vi "Increment Next Column.vi"(11 "SQL Statement in":refnum<class "SQL Statement.lvclass">) -> (3 "SQL Statement out":refnum<class "SQL Statement.lvclass">)   [LabVIEW 2013, in "SQLiteSupport.lvlib" / "SQL Statement.lvclass"]
uses:
  SQL Statement.lvclass
  SQL Statement.lvclass/SQL Statement.ctl
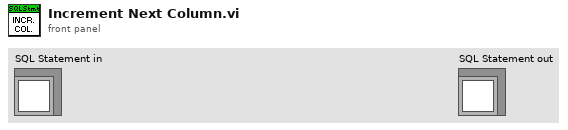
[diagram p1: front panel]
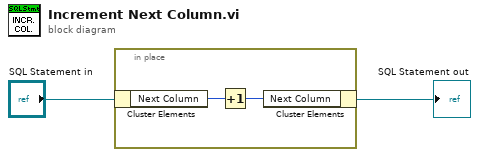
[diagram p0: block diagram]
diagram:
  n1 = in-place {
    n2 = in-place-cluster #1("SQL Statement in") -> ("Next Column"=w4:i32)
    n3 = Increment(x=w4) -> (x+1=w3:i32)
    n4 = in-place-cluster #1("Next Column"=w3) -> (→"SQL Statement out":refnum<class "SQL Statement.lvclass">)
  }
